vi "top_feature-singleImage.vi"() -> ()   [LabVIEW 2015]
uses:
  <vilib>/Utility/file.llb/Write Delimited Spreadsheet (string).vi
  <vilib>/vision/NI_Vision_Development_Module.lvlib
  greenDet.dll
panel:
  in  "单张图像路径":path
  out "Original Image":T1(plugin-control)
  in  "ROI_whole":T2={"Top"=550, "im_height"=1000, "L_left"=650, "im_width"=1050}
  in  "Crop image ?":bool=TRUE
  out "HistStat_whole":dbl[](array[numeric])
  out "AC (Area Convexity)":dbl
  out "P":dbl
  out "TPA (Total projective area)":dbl
  out "SFD":sgl
  out "BW (minimum circumscribed box width)":dbl
  out "BH":dbl
  out "R (Rectangularity)":dbl
  out "IFD":sgl
  out "Hull area":dbl
  out "HWR":dbl
  out "greenDet":dbl
  out "Crop Image":T1(plugin-control)
  out "Binary Image":T1(plugin-control)
  in  "EG threshold":sgl=0.2
  in  "ER threshold":sgl=0.5
  out "GPA (Green projective area)":dbl
  out "YPA (Yellow projective area)":dbl
  out "黄色分量（油菜花）":T1(plugin-control)
  out "黄色分量（油菜花）二值图":T1(plugin-control)
  in  "Pixel Measurements":T3[](array[typedef])=[35] items=["Center of Mass X", "Center of Mass Y", "First Pixel X", "First Pixel Y", "Bounding Rect Left", "Bounding Rect Top", "Bounding Rect Right", "Bounding Rect Bottom", "Max Feret Diameter Start X", "Max Feret Diameter Start Y", "Max Feret Diameter End X", "Max Feret Diameter End Y", "Max Horiz. Segment Length Left", "Max Horiz. Segment Length Right", "Max Horiz. Segment Length Row", "-", "Bounding Rect Width", "Bounding Rect Height", "Bounding Rect Diagonal", "Perimeter", "Convex Hull Perimeter", "Holes' Perimeter", "Max Feret Diameter", "Equivalent Ellipse Major Axis", "Equivalent Ellipse Minor Axis", "Equivalent Ellipse Minor Axis (Feret)", "Equivalent Rect Long Side", "Equivalent Rect Short Side", "Equivalent Rect Diagonal", "Equivalent Rect Short Side (Feret)", "Average Horiz. Segment Length", "Average Vert. Segment Length", "Hydraulic Radius", "Waddel Disk Diameter", "-", "Area", "Holes' Area", "Particle & Holes' Area", "Convex Hull Area", "Image Area", "-", "Number of Holes", "Number of Horiz. Segments", "Number of Vert. Segments", "-", "Orientation", "Max Feret Diameter Orientation", "-", "% Area/Image Area", "% Area/(Particle & Holes' Area)", "Ratio of Equivalent Ellipse Axes", "Ratio of Equivalent Rect Sides", "-", "Elongation Factor", "Compactness Factor", "Heywood Circularity Factor", "Type Factor", "-", "Sum X", "Sum Y", "Sum XX", "Sum XY", "Sum YY", "Sum XXX", "Sum XXY", "Sum XYY", "Sum YYY", "-", "Moment of Inertia XX", "Moment of Inertia XY", "Moment of Inertia YY", "Moment of Inertia XXX", "Moment of Inertia XXY", "Moment of Inertia XYY", "Moment of Inertia YYY", "Norm. Moment of Inertia XX", "Norm. Moment of Inertia XY", "Norm. Moment of Inertia YY", "Norm. Moment of Inertia XXX", "Norm. Moment of Inertia XXY", "Norm. Moment of Inertia XYY", "Norm. Moment of Inertia YYY", "Hu Moment 1", "Hu Moment 2", "Hu Moment 3", "Hu Moment 4", "Hu Moment 5", "Hu Moment 6", "Hu Moment 7"]
  in  "Pixel Measurements 2":T3[](array[typedef])=[35] items=["Center of Mass X", "Center of Mass Y", "First Pixel X", "First Pixel Y", "Bounding Rect Left", "Bounding Rect Top", "Bounding Rect Right", "Bounding Rect Bottom", "Max Feret Diameter Start X", "Max Feret Diameter Start Y", "Max Feret Diameter End X", "Max Feret Diameter End Y", "Max Horiz. Segment Length Left", "Max Horiz. Segment Length Right", "Max Horiz. Segment Length Row", "-", "Bounding Rect Width", "Bounding Rect Height", "Bounding Rect Diagonal", "Perimeter", "Convex Hull Perimeter", "Holes' Perimeter", "Max Feret Diameter", "Equivalent Ellipse Major Axis", "Equivalent Ellipse Minor Axis", "Equivalent Ellipse Minor Axis (Feret)", "Equivalent Rect Long Side", "Equivalent Rect Short Side", "Equivalent Rect Diagonal", "Equivalent Rect Short Side (Feret)", "Average Horiz. Segment Length", "Average Vert. Segment Length", "Hydraulic Radius", "Waddel Disk Diameter", "-", "Area", "Holes' Area", "Particle & Holes' Area", "Convex Hull Area", "Image Area", "-", "Number of Holes", "Number of Horiz. Segments", "Number of Vert. Segments", "-", "Orientation", "Max Feret Diameter Orientation", "-", "% Area/Image Area", "% Area/(Particle & Holes' Area)", "Ratio of Equivalent Ellipse Axes", "Ratio of Equivalent Rect Sides", "-", "Elongation Factor", "Compactness Factor", "Heywood Circularity Factor", "Type Factor", "-", "Sum X", "Sum Y", "Sum XX", "Sum XY", "Sum YY", "Sum XXX", "Sum XXY", "Sum XYY", "Sum YYY", "-", "Moment of Inertia XX", "Moment of Inertia XY", "Moment of Inertia YY", "Moment of Inertia XXX", "Moment of Inertia XXY", "Moment of Inertia XYY", "Moment of Inertia YYY", "Norm. Moment of Inertia XX", "Norm. Moment of Inertia XY", "Norm. Moment of Inertia YY", "Norm. Moment of Inertia XXX", "Norm. Moment of Inertia XXY", "Norm. Moment of Inertia XYY", "Norm. Moment of Inertia YYY", "Hu Moment 1", "Hu Moment 2", "Hu Moment 3", "Hu Moment 4", "Hu Moment 5", "Hu Moment 6", "Hu Moment 7"]
  out "交集像素个数":dbl
  out "交集图":T1(plugin-control)
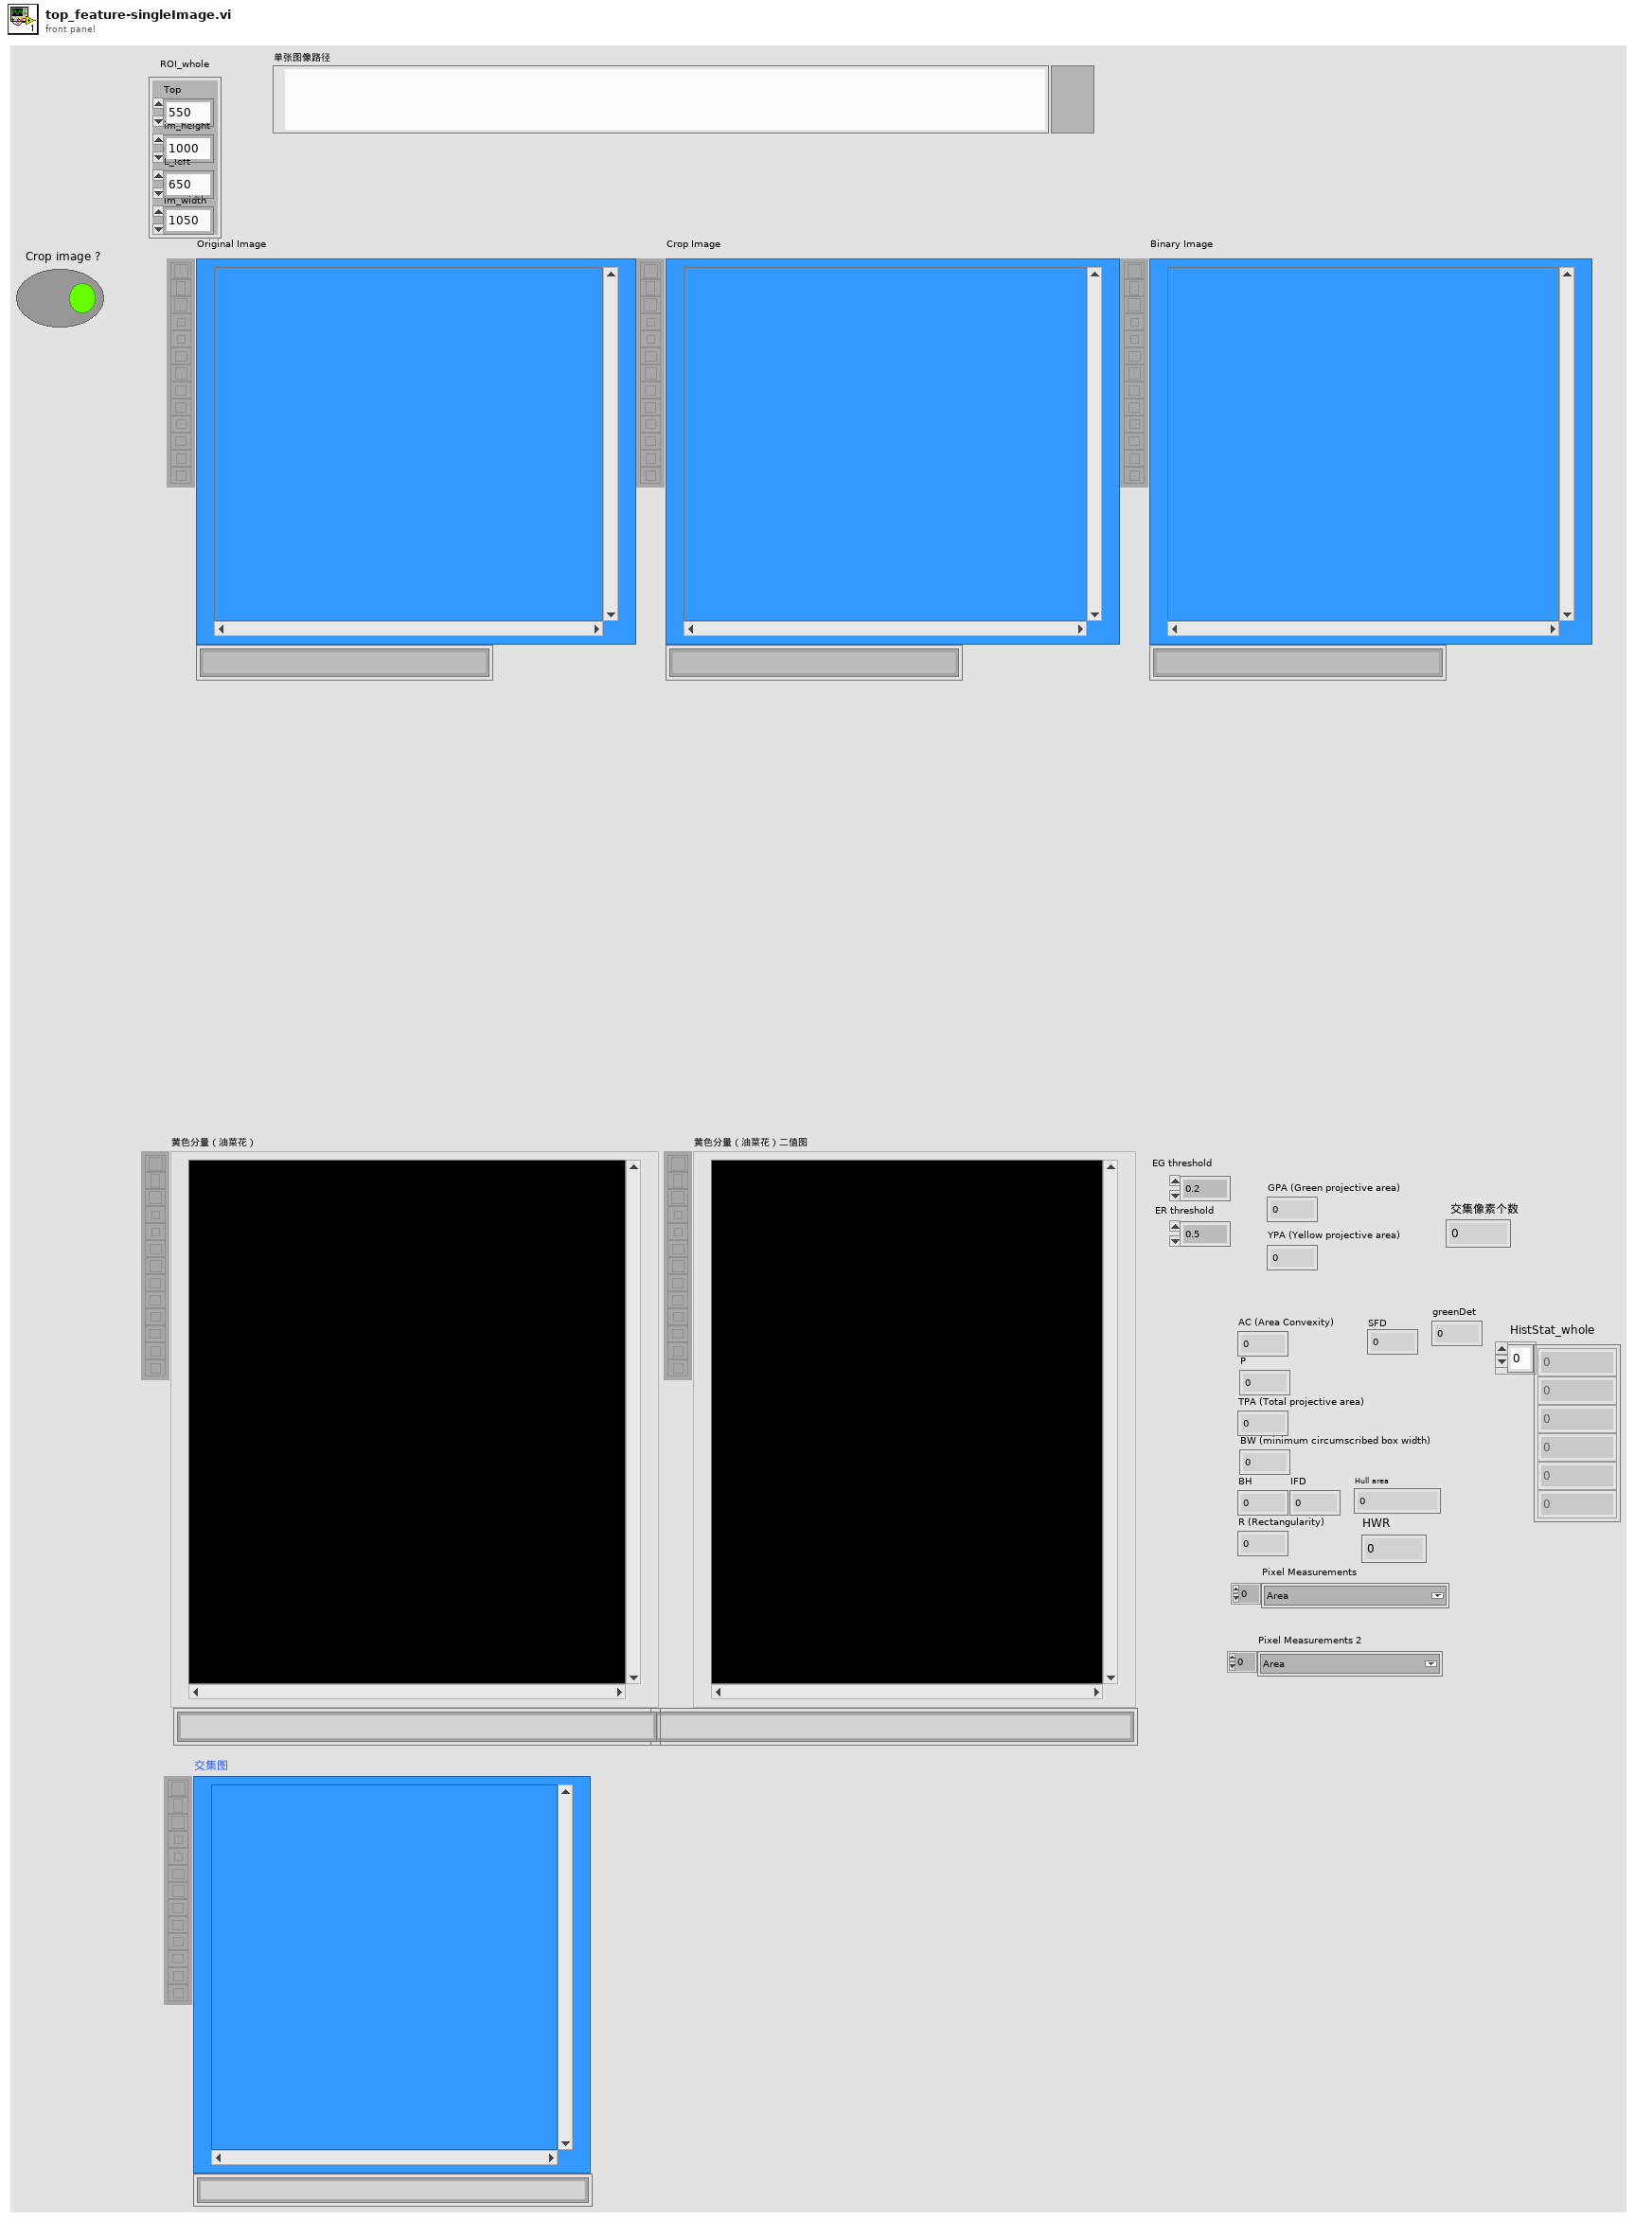
[diagram p1: front panel]
types:
  T1 = typedef "IMAQ Image.ctl" = refnum<image>
  T2 = cluster{"Top":i32, "im_height":i32, "L_left":i32, "im_width":i32}
  T3 = typedef "Particle Parameters" = i32
  T4 = enum32{"AutoM", "Close", "Dilate", "Erode", "Gradient", "Gradient out", "Gradient in", "Hit miss", "Open", "PClose", "POpen", "Thick", "Thin"}
  T5 = typedef "Image Type" = u32
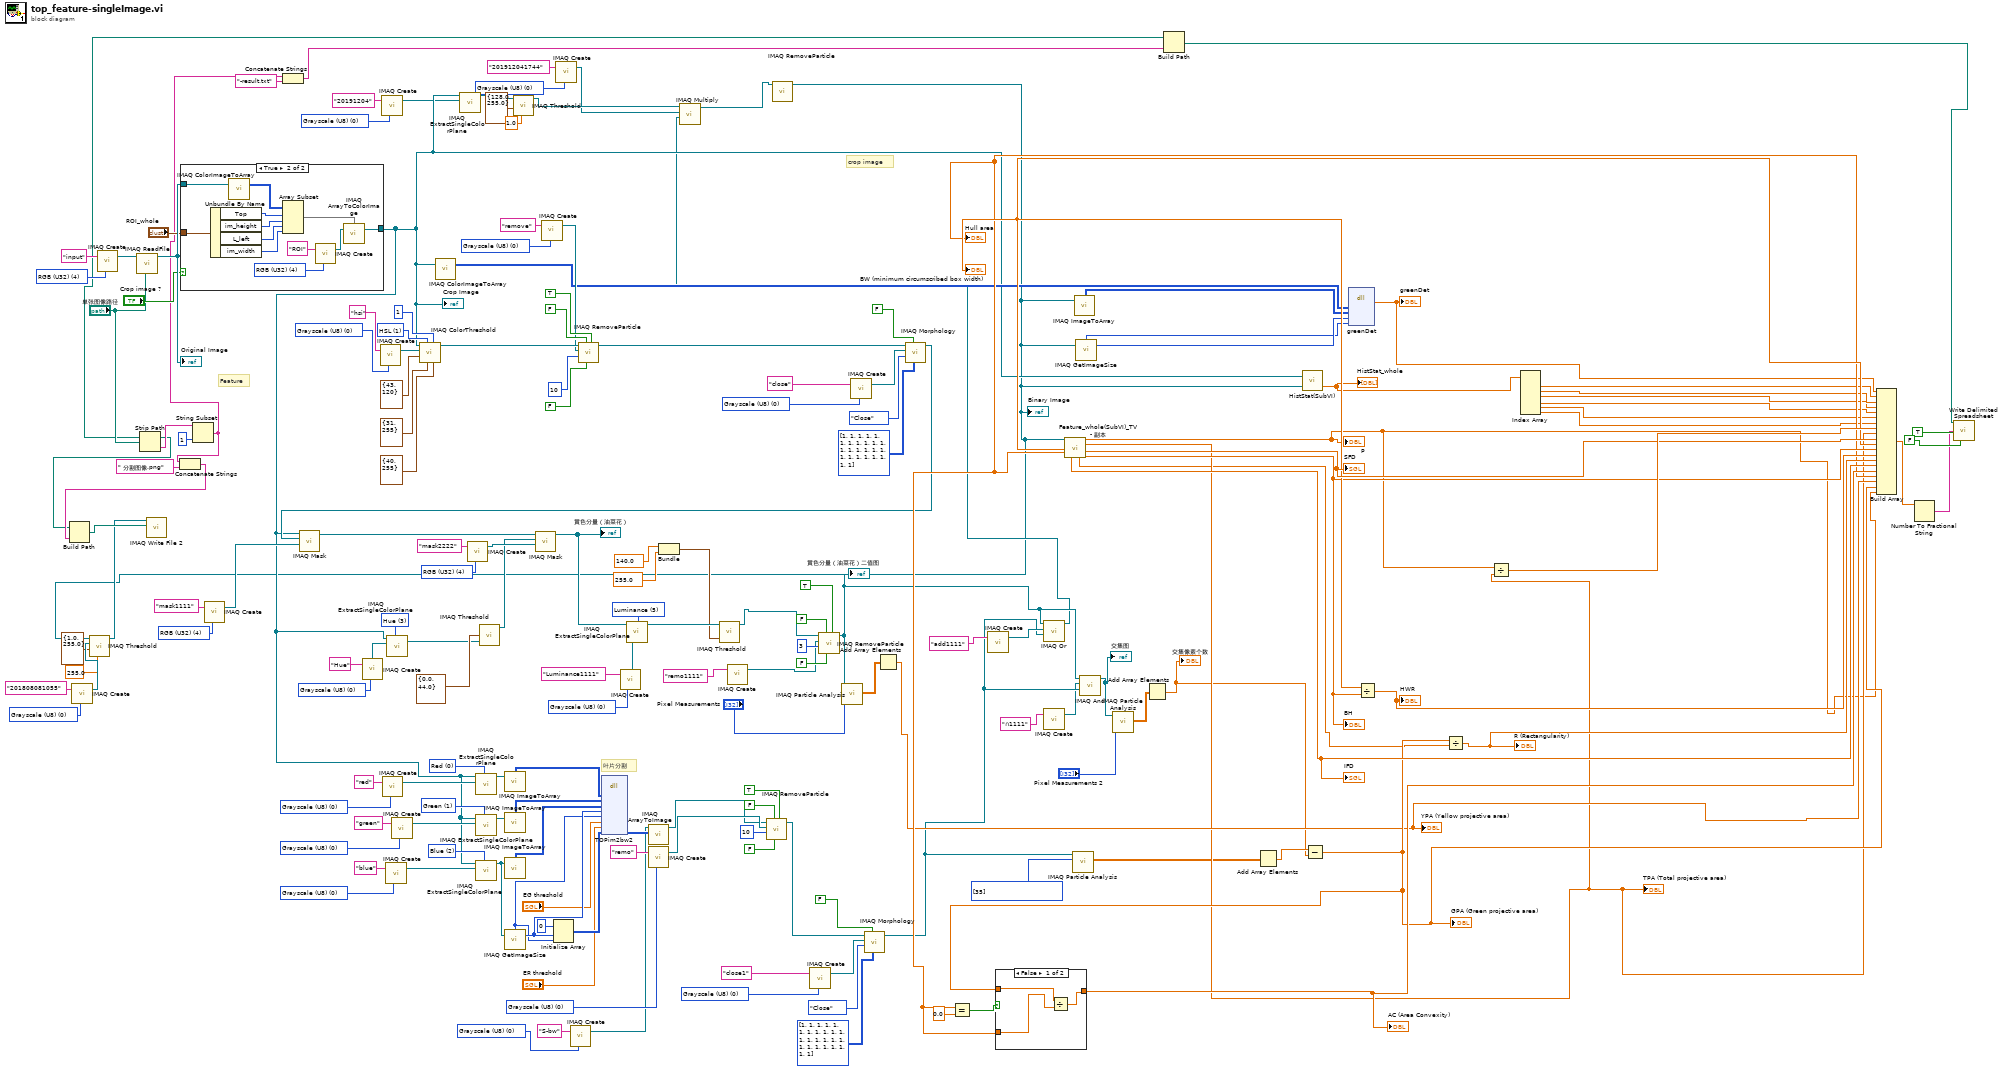
[diagram p0: block diagram]
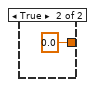
[diagram p2: hidden frame]
diagram:
  w4 = u32 0 items=["Grayscale (U8)", "Grayscale (I16)", "Grayscale (SGL)", "Complex (CSG)", "RGB (U32)", "HSL (U32)", "RGB (U64)"] ("Image Type")
  w13 = u32 0 items=["Grayscale (U8)", "Grayscale (I16)", "Grayscale (SGL)", "Complex (CSG)", "RGB (U32)", "HSL (U32)", "RGB (U64)"] ("Image Type")
  w33 = u32 0 items=["Grayscale (U8)", "Grayscale (I16)", "Grayscale (SGL)", "Complex (CSG)", "RGB (U32)", "HSL (U32)", "RGB (U64)"] ("Image Type")
  w61 = u32 0 items=["Grayscale (U8)", "Grayscale (I16)", "Grayscale (SGL)", "Complex (CSG)", "RGB (U32)", "HSL (U32)", "RGB (U64)"] ("Image Type")
  w64 = 5 items=["Red", "Green", "Blue", "Hue", "Saturation", "Luminance", "Value", "Intensity"] ("Color Plane")
  w68 = u32 0 items=["Grayscale (U8)", "Grayscale (I16)", "Grayscale (SGL)", "Complex (CSG)", "RGB (U32)", "HSL (U32)", "RGB (U64)"] ("Image Type")
  w71 = 3 items=["Red", "Green", "Blue", "Hue", "Saturation", "Luminance", "Value", "Intensity"] ("Color Plane")
  w74 = u32 4 items=["Grayscale (U8)", "Grayscale (I16)", "Grayscale (SGL)", "Complex (CSG)", "RGB (U32)", "HSL (U32)", "RGB (U64)"] ("Image Type")
  w77 = u32 4 items=["Grayscale (U8)", "Grayscale (I16)", "Grayscale (SGL)", "Complex (CSG)", "RGB (U32)", "HSL (U32)", "RGB (U64)"] ("Image Type")
  w86 = u32 0 items=["Grayscale (U8)", "Grayscale (I16)", "Grayscale (SGL)", "Complex (CSG)", "RGB (U32)", "HSL (U32)", "RGB (U64)"] ("Image Type")
  w90 = T3[] [35] items=["Center of Mass X", "Center of Mass Y", "First Pixel X", "First Pixel Y", "Bounding Rect Left", "Bounding Rect Top", "Bounding Rect Right", "Bounding Rect Bottom", "Max Feret Diameter Start X", "Max Feret Diameter Start Y", "Max Feret Diameter End X", "Max Feret Diameter End Y", "Max Horiz. Segment Length Left", "Max Horiz. Segment Length Right", "Max Horiz. Segment Length Row", "-", "Bounding Rect Width", "Bounding Rect Height", "Bounding Rect Diagonal", "Perimeter", "Convex Hull Perimeter", "Holes' Perimeter", "Max Feret Diameter", "Equivalent Ellipse Major Axis", "Equivalent Ellipse Minor Axis", "Equivalent Ellipse Minor Axis (Feret)", "Equivalent Rect Long Side", "Equivalent Rect Short Side", "Equivalent Rect Diagonal", "Equivalent Rect Short Side (Feret)", "Average Horiz. Segment Length", "Average Vert. Segment Length", "Hydraulic Radius", "Waddel Disk Diameter", "-", "Area", "Holes' Area", "Particle & Holes' Area", "Convex Hull Area", "Image Area", "-", "Number of Holes", "Number of Horiz. Segments", "Number of Vert. Segments", "-", "Orientation", "Max Feret Diameter Orientation", "-", "% Area/Image Area", "% Area/(Particle & Holes' Area)", "Ratio of Equivalent Ellipse Axes", "Ratio of Equivalent Rect Sides", "-", "Elongation Factor", "Compactness Factor", "Heywood Circularity Factor", "Type Factor", "-", "Sum X", "Sum Y", "Sum XX", "Sum XY", "Sum YY", "Sum XXX", "Sum XXY", "Sum XYY", "Sum YYY", "-", "Moment of Inertia XX", "Moment of Inertia XY", "Moment of Inertia YY", "Moment of Inertia XXX", "Moment of Inertia XXY", "Moment of Inertia XYY", "Moment of Inertia YYY", "Norm. Moment of Inertia XX", "Norm. Moment of Inertia XY", "Norm. Moment of Inertia YY", "Norm. Moment of Inertia XXX", "Norm. Moment of Inertia XXY", "Norm. Moment of Inertia XYY", "Norm. Moment of Inertia YYY", "Hu Moment 1", "Hu Moment 2", "Hu Moment 3", "Hu Moment 4", "Hu Moment 5", "Hu Moment 6", "Hu Moment 7"] ("Pixel Measurements")
  w124 = T5 0 items=["Grayscale (U8)", "Grayscale (I16)", "Grayscale (SGL)", "Complex (CSG)", "RGB (U32)", "HSL (U32)", "RGB (U64)", "Grayscale (U16)"] ("Image Type")
  w117 = T5 0 items=["Grayscale (U8)", "Grayscale (I16)", "Grayscale (SGL)", "Complex (CSG)", "RGB (U32)", "HSL (U32)", "RGB (U64)", "Grayscale (U16)"] ("Image Type")
  w103 = 2 items=["Red", "Green", "Blue", "Hue", "Saturation", "Luminance", "Value", "Intensity"] ("Color Plane")
  w102 = 0 items=["Red", "Green", "Blue", "Hue", "Saturation", "Luminance", "Value", "Intensity"] ("Color Plane")
  w99 = T5 0 items=["Grayscale (U8)", "Grayscale (I16)", "Grayscale (SGL)", "Complex (CSG)", "RGB (U32)", "HSL (U32)", "RGB (U64)", "Grayscale (U16)"] ("Image Type")
  w97 = 1 items=["Red", "Green", "Blue", "Hue", "Saturation", "Luminance", "Value", "Intensity"] ("Color Plane")
  w94 = T5 0 items=["Grayscale (U8)", "Grayscale (I16)", "Grayscale (SGL)", "Complex (CSG)", "RGB (U32)", "HSL (U32)", "RGB (U64)", "Grayscale (U16)"] ("Image Type")
  w98 = T5 0 items=["Grayscale (U8)", "Grayscale (I16)", "Grayscale (SGL)", "Complex (CSG)", "RGB (U32)", "HSL (U32)", "RGB (U64)", "Grayscale (U16)"] ("Image Type")
  w128 = u32 0 items=["Grayscale (U8)", "Grayscale (I16)", "Grayscale (SGL)", "Complex (CSG)", "RGB (U32)", "HSL (U32)", "RGB (U64)"] ("Image Type")
  w140 = u32 0 items=["Grayscale (U8)", "Grayscale (I16)", "Grayscale (SGL)", "Complex (CSG)", "RGB (U32)", "HSL (U32)", "RGB (U64)"] ("Image Type")
  w143 = u32 0 items=["Grayscale (U8)", "Grayscale (I16)", "Grayscale (SGL)", "Complex (CSG)", "RGB (U32)", "HSL (U32)", "RGB (U64)"] ("Image Type")
  w145 = u16 1 items=["RGB", "HSL", "HSV", "HSI"] ("Color Mode")
  w158 = T5 4 items=["Grayscale (U8)", "Grayscale (I16)", "Grayscale (SGL)", "Complex (CSG)", "RGB (U32)", "HSL (U32)", "RGB (U64)", "Grayscale (U16)"] ("Image Type")
  # "叶片分割"
  # "crop image"
  # "Feature"
  n1 = call "IMAQ Create"("Image Name"="201808081055", "Image Type"=w33) -> ("New Image"=w31:T1)  [unwired: 2 in, 2 out]
  n2 = call "IMAQ Create"("Image Name"="input", "Image Type"=w158) -> ("New Image"=w159:T1)  [unwired: 2 in, 2 out]
  n3 = call "IMAQ ReadFile"("File Path"="单张图像路径", "Image"=w159) -> ("Image Out"=w157:T1)  [unwired: 3 in, 6 out]
  "Original Image" <- w157
  n4 = Strip Path(path="单张图像路径") -> (stripped path=w18:path, name=w24:string)
  n5 = case shown="True" "Crop image ?" {
    tunnel: w157 -> [w182 w189]
    tunnel: "ROI_whole" -> [_ w184]
    tunnel: [w182 w183] -> w14
    frame False {
    }
    frame True {
      w187 = u32 4 items=["Grayscale (U8)", "Grayscale (I16)", "Grayscale (SGL)", "Complex (CSG)", "RGB (U32)", "HSL (U32)", "RGB (U64)"] ("Image Type")
      n6 = Unbundle By Name(w184) -> ("Top"=w191:i32, "im_height"=w192:i32, "L_left"=w193:i32, "im_width"=w194:i32)
      n7 = call "IMAQ ColorImageToArray"("Image"=w189) -> ("Image Pixels (U32)"=w190:u32[][])  [unwired: 2 in, 3 out]
      n8 = Array Subset(array=w190, index (row)=w191, length (row)=w192, index (col)=w193, length (col)=w194) -> (w185:u32[][])
      n9 = call "IMAQ Create"("Image Name"="ROI", "Image Type"=w187) -> ("New Image"=w186:T1)  [unwired: 2 in, 2 out]
      n10 = call "IMAQ ArrayToColorImage"("Image Pixels (U32)"=w185, "Image"=w186) -> ("Image Out"=w183:T1)  [unwired: 2 in, 2 out]
    }
  }
  "Crop Image" <- w14
  n11 = String Subset(string=w24, length (rest)=1 ("length (rest)")) -> (substring=w20:string)  [unwired: 1 in]
  n12 = Concatenate Strings(w20, " 分割图像.png" ("string")) -> (w21:string)
  n13 = Build Path(base path=w18, name or relative path=w21) -> (appended path=w34:path)
  n14 = call "IMAQ Create"("Image Name"="mask1111", "Image Type"=w77) -> ("New Image"=w76:T1)  [unwired: 2 in, 2 out]
  n15 = Concatenate Strings(w20, "-result.txt" ("string")) -> (w17:string)
  n16 = call "IMAQ Create"("Image Name"="Hue", "Image Type"=w68) -> ("New Image"=w67:T1)  [unwired: 2 in, 2 out]
  n17 = call "IMAQ Create"("Image Name"="hsi", "Image Type"=w143) -> ("New Image"=w142:T1)  [unwired: 2 in, 2 out]
  n18 = call "IMAQ Create"("Image Name"="20191204", "Image Type"=w13) -> ("New Image"=w11:T1)  [unwired: 2 in, 2 out]
  n19 = call "IMAQ Create"("Image Name"="red", "Image Type"=w98) -> ("New Image"=w93:T1)  [unwired: 2 in, 2 out]
  n20 = call "IMAQ Create"("Image Name"="blue", "Image Type"=w94) -> ("New Image"=w96:T1)  [unwired: 2 in, 2 out]
  n21 = call "IMAQ ExtractSingleColorPlane"("Color Plane"=w71, "Image Dst"=w67, "Image Src"=w14) -> ("Image Dst Out"=w69:T1)  [unwired: 1 in, 7 out]
  n22 = call "IMAQ Create"("Image Name"="green", "Image Type"=w99) -> ("New Image"=w101:T1)  [unwired: 2 in, 2 out]
  n23 = call "IMAQ ColorThreshold"("Blue or Luma or Val or Inten Range"=cluster{"Lower value":i32, "Upper value":i32} {"Lower value"=40, "Upper value"=255}, "Replace Value"=1, "Green or Sat Range"=cluster{"Lower value":i32, "Upper value":i32} {"Lower value"=31, "Upper value"=255}, "Color Mode"=w145, "Red or Hue Range"=cluster{"Lower value":i32, "Upper value":i32} {"Lower value"=43, "Upper value"=120}, "Image Dst"=w142, "Image Src"=w14) -> ("Image Dst Out"=w146:T1)  [unwired: 1 in, 3 out]
  n24 = call "IMAQ ColorImageToArray"("Image"=w14) -> ("Image Pixels (U32)"=w138:u32[][])  [unwired: 2 in, 3 out]
  n25 = call "IMAQ ExtractSingleColorPlane"("Image Dst"=w11, "Image Src"=w14) -> ("Image Dst Out"=w10:T1)  [unwired: 8 in, 1 out]
  n26 = call "IMAQ Create"("Image Name"="mask2222", "Image Type"=w74) -> ("New Image"=w73:T1)  [unwired: 2 in, 2 out]
  n27 = call "IMAQ ExtractSingleColorPlane"("Color Plane"=w102, "Image Dst"=w93, "Image Src"=w14) -> ("Image Dst Out"=w105:T1)  [unwired: 1 in, 7 out]
  n28 = call "IMAQ ExtractSingleColorPlane"("Color Plane"=w97, "Image Dst"=w101, "Image Src"=w14) -> ("Image Dst Out"=w104:T1)  [unwired: 1 in, 7 out]
  n29 = call "IMAQ ExtractSingleColorPlane"("Color Plane"=w103, "Image Dst"=w96, "Image Src"=w14) -> ("Image Dst Out"=w109:T1)  [unwired: 1 in, 7 out]
  n30 = call "IMAQ Threshold"("Range"=cluster{"Lower value":sgl, "Upper value":sgl} {"Lower value"=0.0, "Upper value"=44.0}, "Image Src"=w69) -> ("Image Dst Out"=w47:T1)  [unwired: 4 in, 5 out]
  n31 = call "IMAQ ImageToArray"("Image"=w105) -> ("Image Pixels (U8)"=w107:u8[][])  [unwired: 2 in, 5 out]
  n32 = call "IMAQ ImageToArray"("Image"=w104) -> ("Image Pixels (U8)"=w106:u8[][])  [unwired: 2 in, 5 out]
  n33 = call "IMAQ ImageToArray"("Image"=w109) -> ("Image Pixels (U8)"=w108:u8[][])  [unwired: 2 in, 5 out]
  n34 = call "IMAQ GetImageSize"("Image"=w109) -> ("Y Resolution"=w114:i32, "X Resolution"=w113:i32)  [unwired: 1 in, 3 out]
  n35 = call "IMAQ Threshold"("Replace Value"=sgl 1.0, "Range"=cluster{"Lower value":sgl, "Upper value":sgl} {"Lower value"=128.0, "Upper value"=255.0}, "Image Src"=w10) -> ("Image Dst Out"=w7:T1)  [unwired: 7 in, 1 out]
  n36 = call "IMAQ Create"("Image Name"="remove", "Image Type"=w140) -> ("New Image"=w139:T1)  [unwired: 2 in, 2 out]
  n37 = Initialize Array(u8 0 ("element"), w114, w113) -> (w115:u8[][])
  n38 = call "IMAQ Create"("Image Name"="201912041744", "Image Type"=w4) -> ("New Image"=w3:T1)  [unwired: 2 in, 2 out]
  n39 = call "IMAQ Create"("Image Name"="S-bw", "Image Type"=w117) -> ("New Image"=w118:T1)  [unwired: 2 in, 2 out]
  n40 = call "IMAQ RemoveParticle"("Connectivity 4/8 (8)"=TRUE, "Low Pass/High Pass (Low)"=FALSE, "Square/Hexa (Square)"=FALSE, "Number of Erosion"=10, "Image Dst"=w139, "Image Src"=w146) -> ("Image Dst Out"=w130:T1)  [unwired: 1 in, 4 out]
  n41 = dll-call lib="PTH2¢abs Dfhä¼ è¾E\tRPAE Workæç®éè¯»æ²¹è æç«  ææµ·æ¶ææµ·æ¶oilseedRape measurement proceduresæ²¹èé¡¶è§d..." fn="TOPim2bw2"("R"=w107, "G"=w106, "B"=w108, "row"=w114, "col"=w113, "EGthreshold"="EG threshold", "ERthreshold"="ER threshold", "bw"=w115) -> ("bw"=w119:u8[][])  [unwired: 10 in, 3 out]
  n42 = call "IMAQ Create"("Image Name"="Luminance1111", "Image Type"=w61) -> ("New Image"=w63:T1)  [unwired: 2 in, 2 out]
  n43 = call "IMAQ ArrayToImage"("Image Pixels (U8)"=w119, "Image"=w118) -> ("Image Out"=w83:T1)  [unwired: 4 in, 5 out]
  n44 = call "IMAQ Create"("Image Name"="remo", "Image Type"=w124) -> ("New Image"=w126:T1)  [unwired: 2 in, 2 out]
  n45 = Bundle("Lower value"=sgl 140.0, "Upper value"=sgl 255.0) -> (w57:cluster{"Lower value":sgl, "Upper value":sgl})  [unwired: 1 in]
  n46 = call "IMAQ Create"("Image Name"="remo1111") -> ("New Image"=w50:T1)  [unwired: 3 in, 2 out]
  n47 = call "IMAQ RemoveParticle"("Connectivity 4/8 (8)"=TRUE, "Low Pass/High Pass (Low)"=FALSE, "Square/Hexa (Square)"=FALSE, "Number of Erosion"=10, "Image Dst"=w126, "Image Src"=w83) -> ("Image Dst Out"=w82:T1)  [unwired: 1 in, 4 out]
  n48 = call "IMAQ Create"("Image Name"="close1", "Image Type"=w86) -> ("New Image"=w85:T1)  [unwired: 2 in, 2 out]
  n49 = call "IMAQ Create"("Image Name"="close", "Image Type"=w128) -> ("New Image"=w127:T1)  [unwired: 2 in, 2 out]
  n50 = call "IMAQ Morphology"("Structuring Element"=i32[][] [[1, 1, 1, 1, 1], [1, 1, 1, 1, 1], [1, 1, 1, 1, 1], [1, 1, 1, 1, 1], [1, 1, 1, 1, 1]], "Square/Hexa (Square)"=FALSE, "Operation"=T4."Close", "Image Dst"=w85, "Image Src"=w82) -> ("Image Dst Out"=w42:T1)  [unwired: 2 in, 4 out]
  n51 = call "IMAQ Morphology"("Structuring Element"=i32[][] [[1, 1, 1, 1, 1], [1, 1, 1, 1, 1], [1, 1, 1, 1, 1], [1, 1, 1, 1, 1], [1, 1, 1, 1, 1]], "Square/Hexa (Square)"=FALSE, "Operation"=T4."Close", "Image Dst"=w127, "Image Src"=w130) -> ("Image Dst Out"=w45:T1)  [unwired: 2 in, 4 out]
  n52 = call "IMAQ Mask"("Image Dst"=w76, "Image Mask"=w45, "Image Src"=w14) -> ("Image Dst Out"=w72:T1)  [unwired: 1 in, 2 out]
  n53 = call "IMAQ Mask"("Image Dst"=w73, "Image Mask"=w47, "Image Src"=w72) -> ("Image Dst Out"=w62:T1)  [unwired: 1 in, 2 out]
  "黄色分量（油菜花）" <- w62
  n54 = call "IMAQ ExtractSingleColorPlane"("Color Plane"=w64, "Image Dst"=w63, "Image Src"=w62) -> ("Image Dst Out"=w65:T1)  [unwired: 1 in, 7 out]
  n55 = call "IMAQ Threshold"("Range"=w57, "Image Src"=w65) -> ("Image Dst Out"=w49:T1)  [unwired: 4 in, 5 out]
  n56 = call "IMAQ RemoveParticle"("Connectivity 4/8 (8)"=TRUE, "Low Pass/High Pass (Low)"=FALSE, "Square/Hexa (Square)"=FALSE, "Number of Erosion"=3, "Image Dst"=w50, "Image Src"=w49) -> ("Image Dst Out"=w43:T1)  [unwired: 1 in, 4 out]
  "黄色分量（油菜花）二值图" <- w43
  n57 = call "IMAQ Particle Analysis"("Pixel Measurements"="Pixel Measurements", "Image"=w43) -> ("Particle Measurements (Pixels)"=w56:dbl[][])  [unwired: 3 in, 6 out]
  n58 = Add Array Elements(numeric array=w56) -> (sum=w163:dbl)
  "YPA (Yellow projective area)" <- w163
  n59 = call "IMAQ Create"("Image Name"="add1111") -> ("New Image"=w44:T1)  [unwired: 3 in, 2 out]
  n60 = call "IMAQ Or"("Image Src B"=w42, "Image Dst"=w44, "Image Src A"=w43) -> ("Image Dst Out"=w6:T1)  [unwired: 7 in, 1 out]
  n61 = call "IMAQ Multiply"("Image Src A"=w7, "Image Dst"=w3, "Image Src B"=w6) -> ("Image Dst Out"=w2:T1)  [unwired: 4 in, 1 out]
  n62 = call "IMAQ RemoveParticle"("Image Src"=w2) -> ("Image Dst Out"=w1:T1)  [unwired: 6 in, 4 out]
  "Binary Image" <- w1
  n63 = call "IMAQ Threshold"("Replace Value"=sgl 255.0, "Range"=cluster{"Lower value":sgl, "Upper value":sgl} {"Lower value"=1.0, "Upper value"=255.0}, "Image Dst"=w31, "Image Src"=w1) -> ("Image Dst Out"=w28:T1)  [unwired: 6 in, 1 out]
  n64 = call-poly "IMAQ Write File 2"("File Path"=w34, "Image"=w28) -> ()  [unwired: 8 in, 2 out]
  n65 = call "IMAQ Create"("Image Name"="∩1111") -> ("New Image"=w40:T1)  [unwired: 3 in, 2 out]
  n66 = call "Feature_whole(SubVI)_TV - 副本.vi"("Binary Image"=w1) -> ("P"=w161:dbl, "SA"=w162:dbl, "SFD"=w180:sgl, "Hull area"=w173:dbl, "SW"=w179:dbl, "IFD"=w175:sgl, "最小外接矩面积"=w81:dbl, "SH"=w178:dbl)  [unwired: 6 in, 1 out]
  "P" <- w161
  "TPA (Total projective area)" <- w162
  "SFD" <- w180
  "BW (minimum circumscribed box width)" <- w179
  "BH" <- w178
  "IFD" <- w175
  "Hull area" <- w173
  n67 = Equal?(x=w173, y=0.0) -> (x = y?=w80:bool)
  n68 = call "IMAQ Particle Analysis"("Pixel Measurements"=w90, "Image"=w42) -> ("Particle Measurements (Pixels)"=w91:dbl[][])  [unwired: 3 in, 6 out]
  n69 = call "IMAQ ImageToArray"("Image"=w1) -> ("Image Pixels (U8)"=w137:u8[][])  [unwired: 2 in, 5 out]
  n70 = call "IMAQ GetImageSize"("Image"=w1) -> ("Y Resolution"=w136:i32, "X Resolution"=w135:i32)  [unwired: 1 in, 3 out]
  n71 = call "IMAQ And"("Image Src B"=w42, "Image Dst"=w40, "Image Src A"=w43) -> ("Image Dst Out"=w36:T1)  [unwired: 7 in, 1 out]
  "交集图" <- w36
  n72 = call "IMAQ Particle Analysis"("Pixel Measurements"="Pixel Measurements 2", "Image"=w36) -> ("Particle Measurements (Pixels)"=w39:dbl[][])  [unwired: 3 in, 6 out]
  n73 = Add Array Elements(numeric array=w39) -> (sum=w35:dbl)
  "交集像素个数" <- w35
  n74 = Build Path(base path=w18, name or relative path=w17) -> (appended path=w16:path)
  n75 = Add Array Elements(numeric array=w91) -> (sum=w37:dbl)
  n76 = call "HistStat(SubVI).vi"("Binary Image"=w1, "Original Image"=w14) -> ("HistStat"=w134:dbl[])  [unwired: 1 out]
  "HistStat_whole" <- w134
  n77 = Subtract(x=w37, y=w35) -> (x-y=w164:dbl)
  "GPA (Green projective area)" <- w164
  n78 = case shown="False" w80 {
    tunnel: w164 -> [w197 _]
    tunnel: w173 -> [w196 _]
    tunnel: [w195 0.0] -> w174
    frame False {
      n79 = Divide(x=w197, y=w196) -> (x/y=w195:dbl)
    }
    frame True {
    }
  }
  "AC (Area Convexity)" <- w174
  n80 = dll-call lib="PTH2abs Dfhä¼ è¾E\tRPAE Workæç®éè¯»æ²¹è æç«  ææµ·æ¶ææµ·æ¶oilseedRape measurement proceduresæ²¹èé¡¶è§top_featuresgreenDet.dll" fn="greenDet"("oriArray"=w138, "binArray"=w137, "imageRows"=w136, "imageCols"=w135) -> ("greenDet"=w172:dbl)  [unwired: 7 in, 2 out]
  "greenDet" <- w172
  n81 = Divide(x=w179, y=w178) -> (x/y=w177:dbl)
  "HWR" <- w177
  n82 = Divide(x=w164, y=w81) -> (x/y=w176:dbl)
  "R (Rectangularity)" <- w176
  n83 = Divide(x=w161, y=w162) -> (x/y=w181:dbl)
  n84 = Index Array(array=w134) -> (element #1=w171:dbl, element #2=w170:dbl, element #3=w169:dbl, element #4=w168:dbl, element #5=w167:dbl, element #6=w166:dbl)  [unwired: 6 in]
  n85 = Build Array(w172, w171, w170, w169, w168, w167, w166, w181, w162, w180, w179, w178, w177, w176, w175, w174, w173, w163, w164, w161) -> (w26:dbl[])
  n86 = Number To Fractional String(number=w26) -> (F-format string=w15:string[])  [unwired: 3 in]
  n87 = call-poly <vilib>:"Write Delimited Spreadsheet.vi"("file path (dialog if empty)"=w16, "1D data"=w15, "append to file? (F)"=TRUE, "transpose? (F)"=FALSE ("append to file? (new file:F)")) -> ()  [unwired: 10 in, 2 out]
